vi "NetworkUDP_Close.vi"(8 "error in (no error)":errorcluster, 11 "UDP Network Connection in":refnum<k16>) -> (0 "error out":errorcluster)   [LabVIEW 2019, in "Trajectory_Library.lvlib"]
doc: "Close an open UDP connection.\n\nInputs\n -- UDP Network Connection -- UDP Connection Reference -- The connection to clost\n -- Error in -- Error cluster -- input propagated error. (Optional. Default: No error )\n\nOutputs:\n -- Error out -- Error cluster -- output propagated error."
uses:
  Trajectory_Library.lvlib
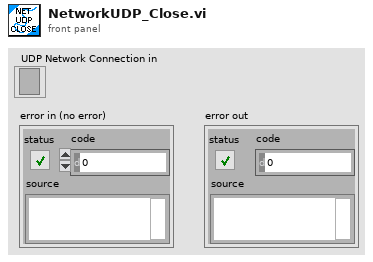
[diagram p1: front panel]
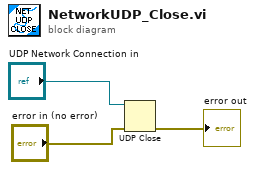
[diagram p0: block diagram]
diagram:
  n1 = UDP Close(connection ID="UDP Network Connection in", 8:"error in (no error)") -> (error out=→"error out":errorcluster)  [unwired: 1 out]
